vi "2012_01_17 Pre-Clinical Crunch.vi"(8 "error in (no error)":errorcluster, 9 "data":waveform(dbl)[](array[waveform]), 10 "Elapsed Time (s)":dbl, 11 "cluster":T1) -> (0 "error out":errorcluster, 2 "Dynamic Data Type":dynamicdata(waveform), 3 "Motor Out":T2={"Fail"=FALSE, "RPM"=0, "Supply (V)"=0.0, "Time"=1.0, "Counter"=0.0, "Torque (mNm)"=0.0, "Electrical (W)"=0.0, "Motor Eff"=0.0, "Mechanical (W)"=0.0, "Supply (W)"=0.0, "ESC Eff"=0.0} {"ESC Eff" format="%#_3g%%"; "Supply (W)" format="%.3f"; "Mechanical (W)" format="%.3f"; "Motor Eff" format="%#_3g%%"; "Electrical (W)" format="%.3f"; "Torque (mNm)" format="%.3f"; "Time" format="%<%H:%M:%S>t"; "Supply (V)" format="%.2f"})   [LabVIEW 2013]
uses:
  Pre-Clinical Type Def.ctl
  <vilib>/measure/matone.llb/Extract Single Tone Information 1 Chan.vi
  <vilib>/measure/madcrms.llb/Basic Averaged DC-RMS for 1 Chan.vi
  <vilib>/express/express arith-compare/Formula/XNode/ExpressFormulaBlockNode.xnode
  <vilib>/measure/NI_MAPro.lvlib
panel:
  # "Stopped"
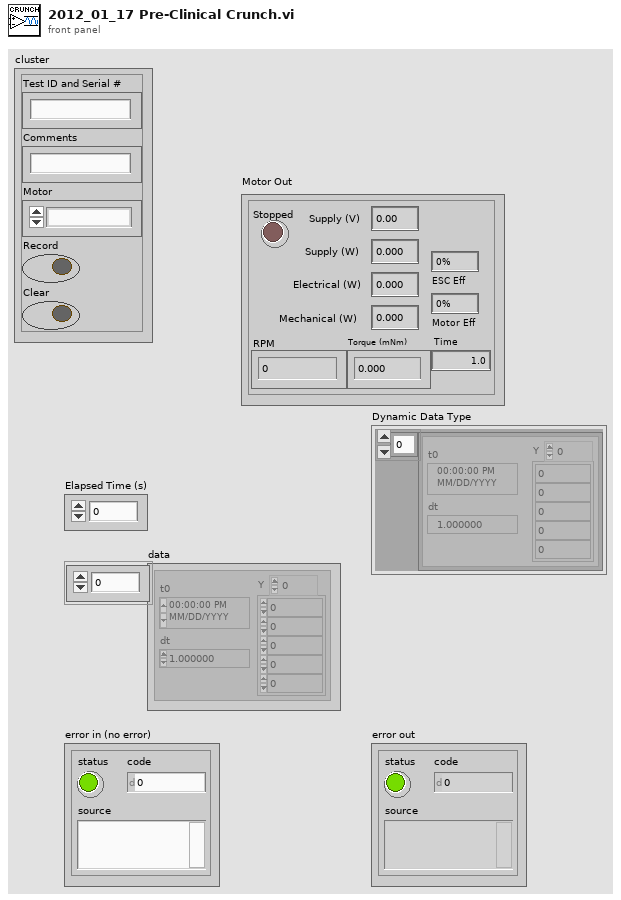
[diagram p1: front panel]
types:
  T1 = cluster{"Test ID and Serial #":string, "Comments":string, "Motor":enum16{"", "Maxon EC6 6V", "Maxon EC4 6V", "FH 0620 6V", "FH 0620 12V", "FH 0427 6V K2540"}, "Record":bool, "Clear":bool}
  T2 = typedef "Pre-Clinical Type Def.ctl" = cluster{"Fail":bool, "RPM":u64, "Supply (V)":dbl, "Time":dbl, "Counter":dbl, "Torque (mNm)":dbl, "Electrical (W)":dbl, "Motor Eff":dbl, "Mechanical (W)":dbl, "Supply (W)":dbl, "ESC Eff":dbl}
  T3 = enum16{"", "Maxon EC6 6V", "Maxon EC4 6V", "FH 0620 6V", "FH 0620 12V", "FH 0427 6V K2540"}
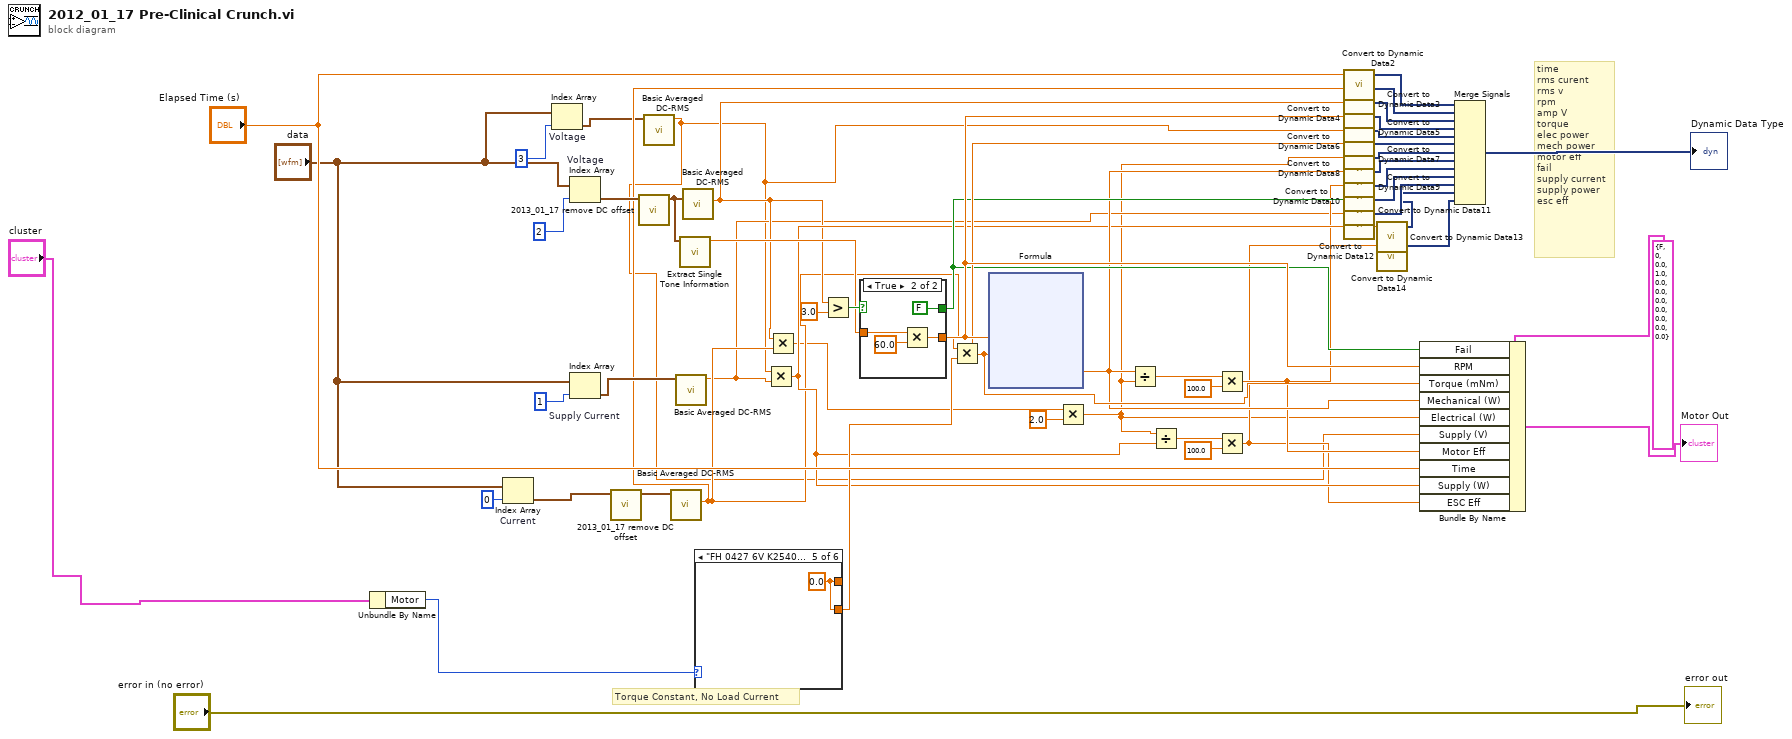
[diagram p0: block diagram]
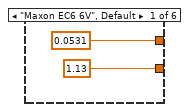
[diagram p2: hidden frame]
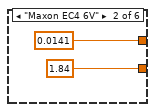
[diagram p3: hidden frame]
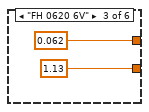
[diagram p4: hidden frame]
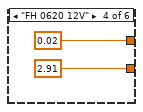
[diagram p5: hidden frame]
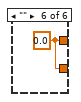
[diagram p6: hidden frame]
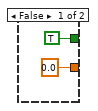
[diagram p7: hidden frame]
diagram:
  # "time\nrms curent\nrms v\nrpm\namp V\ntorque\nelec power\nmech power\nmotor eff\nfail\nsupply current\nsupply power\nesc eff"
  # "Torque Constant, No Load Current"
  n1 = Unbundle By Name("cluster") -> ("Motor"=w47:T3)
  n2 = Index Array "Current"(array="data", index=0) -> (element=w32:waveform(dbl))
  n3 = Index Array "Voltage"(array="data", index=3 ("y")) -> (element=w5:waveform(dbl))
  n4 = Index Array "Voltage"(array="data", index=2 ("y")) -> (element=w30:waveform(dbl))
  n5 = Index Array "Supply Current"(array="data", index=1) -> (element=w27:waveform(dbl))
  n6 = call "2013_01_17 remove DC offset.vi"("Waveform in"=w32) -> ("Waveform out"=w31:waveform(dbl))  [unwired: 10 in]
  n7 = call "2013_01_17 remove DC offset.vi"("Waveform in"=w30) -> ("Waveform out"=w29:waveform(dbl))  [unwired: 10 in]
  n8 = call-poly <vilib>:"Basic Averaged DC-RMS.vi"("signal in"=w5) -> ("DC value"=w4:dbl)  [unwired: 7 in, 3 out]
  n9 = call-poly <vilib>:"Basic Averaged DC-RMS.vi"("signal in"=w31) -> ("RMS value"=w14:dbl)  [unwired: 7 in, 3 out]
  n10 = call-poly <vilib>:"Basic Averaged DC-RMS.vi"("signal in"=w27) -> ("DC value"=w11:dbl)  [unwired: 7 in, 3 out]
  n11 = call-poly <vilib>:"Extract Single Tone Information.vi"("time signal in"=w29) -> ("detected frequency"=w48:dbl)  [unwired: 5 in, 5 out]
  n12 = call-poly <vilib>:"Basic Averaged DC-RMS.vi"("signal in"=w29) -> ("RMS value"=w15:dbl)  [unwired: 7 in, 3 out]
  n13 = case shown="\"FH 0427 6V K2540\"" w47 {
    tunnel: [1.13 1.84 1.13 2.91 w62 w63] -> w26
    tunnel: [0.0531 0.0141 0.062 0.02 w62 w63] -> _
    frame "Maxon EC6 6V", Default {
    }
    frame "Maxon EC4 6V" {
    }
    frame "FH 0620 6V" {
    }
    frame "FH 0620 12V" {
    }
    frame "FH 0427 6V K2540" {
      w62 = 0.0
    }
    frame "" {
      w63 = 0.0
    }
  }
  n14 = Multiply(x=w4, y=w11) -> (x*y=w22:dbl)
  n15 = Multiply(x=w15, y=w14) -> (x*y=w10:dbl)
  n16 = Greater?(x=w15, y=3.0) -> (0:w50:bool)
  n17 = case shown="True" w50 {
    tunnel: [0.0 ("y") w69] -> w46
    tunnel: w48 -> [_ w67]
    tunnel: [TRUE FALSE] -> w34
    frame False {
    }
    frame True {
      n18 = Multiply(x=w67, y=60.0) -> (x*y=w69:dbl)
    }
  }
  n19 = Multiply(x=w14, y=w26) -> (x*y=w45:dbl)
  n20 = xnode "Formula"("RPM"=w46, "Torque"=w45) -> ("Result"=w23:dbl)  [unwired: 1 in, 1 out]
  n21 = Multiply(x=w10, y=2.0) -> (x*y=w8:dbl)
  n22 = Divide(x=w23, y=w8) -> (x/y=w19:dbl)
  n23 = Divide(x=w8, y=w22) -> (x/y=w17:dbl)
  n24 = Multiply(x=w19, y=100.0) -> (x*y=w18:dbl)
  n25 = Multiply(x=w17, y=100.0) -> (x*y=w16:dbl)
  n26 = call "Convert to Dynamic Data2"("Double"="Elapsed Time (s)") -> ("Dynamic Data Type"=w44:dynamicdata)  [unwired: 3 in]
  n27 = call "Convert to Dynamic Data3"("Double"=w14) -> ("Dynamic Data Type"=w43:dynamicdata)  [unwired: 3 in]
  n28 = call "Convert to Dynamic Data4"("Double"=w15) -> ("Dynamic Data Type"=w42:dynamicdata)  [unwired: 3 in]
  n29 = call "Convert to Dynamic Data5"("Double"=w46) -> ("Dynamic Data Type"=w41:dynamicdata)  [unwired: 3 in]
  n30 = call "Convert to Dynamic Data6"("Double"=w4) -> ("Dynamic Data Type"=w40:dynamicdata)  [unwired: 3 in]
  n31 = call "Convert to Dynamic Data7"("Double"=w45) -> ("Dynamic Data Type"=w39:dynamicdata)  [unwired: 3 in]
  n32 = call "Convert to Dynamic Data8"("Double"=w8) -> ("Dynamic Data Type"=w38:dynamicdata)  [unwired: 3 in]
  n33 = call "Convert to Dynamic Data9"("Double"=w23) -> ("Dynamic Data Type"=w37:dynamicdata)  [unwired: 3 in]
  n34 = call "Convert to Dynamic Data10"("Double"=w18) -> ("Dynamic Data Type"=w36:dynamicdata)  [unwired: 3 in]
  n35 = call "Convert to Dynamic Data11"("Boolean"=w34) -> ("Dynamic Data Type"=w35:dynamicdata)  [unwired: 3 in]
  n36 = call "Convert to Dynamic Data12"("Double"=w11) -> ("Dynamic Data Type"=w33:dynamicdata)  [unwired: 3 in]
  n37 = call "Convert to Dynamic Data13"("Double"=w22) -> ("Dynamic Data Type"=w25:dynamicdata)  [unwired: 3 in]
  n38 = call "Convert to Dynamic Data14"("Double"=w16) -> ("Dynamic Data Type"=w24:dynamicdata)  [unwired: 3 in]
  n39 = Bundle By Name(cluster=T2 {"Fail"=FALSE, "RPM"=0, "Supply (V)"=0.0, "Time"=1.0, "Counter"=0.0, "Torque (mNm)"=0.0, "Electrical (W)"=0.0, "Motor Eff"=0.0, "Mechanical (W)"=0.0, "Supply (W)"=0.0, "ESC Eff"=0.0} ("Motor Out"), "Fail"=w34, "RPM"=w46, "Torque (mNm)"=w45, "Mechanical (W)"=w23, "Electrical (W)"=w8, "Supply (V)"=w4, "Motor Eff"=w18, "Time"="Elapsed Time (s)", "Supply (W)"=w22, "ESC Eff"=w16) -> (→"Motor Out":T2)
  n40 = Merge Signals(w44, w43, w42, w41, w40, w39, w38, w37, w36, w35, w33, w25, w24) -> (→"Dynamic Data Type":dynamicdata)
  "error out" <- "error in (no error)"
